vi "Estructuras de Datos.vi"() -> ()   [LabVIEW 2020]
panel:
  in  "Knob":dbl(knob) scale=0.0..100.0
  out "Thermometer":dbl(slide) scale=0.0..100.0
  # "Indicador"
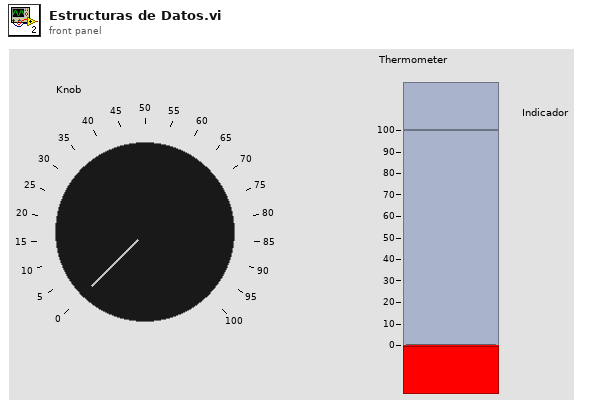
[diagram p1: front panel]
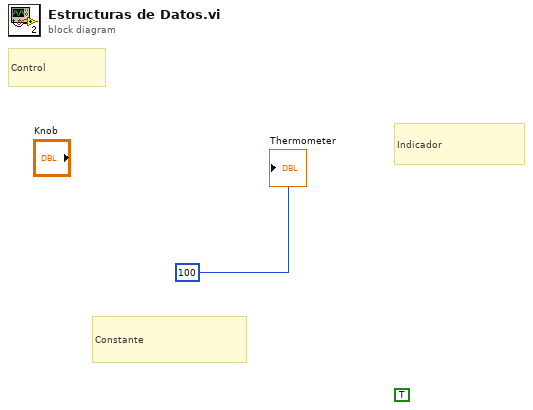
[diagram p0: block diagram]
diagram:
  (unwired) TRUE
  # "Constante"
  # "Control"
  # "Indicador"
  "Thermometer" <- 100
